vi "Compute Spot Pattern v2.vi"(0 "Images Dest":T1, 2 "Pattern Definition":T4={"X pitch"=20.0, "rotation"=0.0, "Center H"=0.0, "Center V"=0.0, "# Spots H"=8, "# Spots V"=8, "Spot size"=20.0, "ref_spot _dark"=FALSE, "Exact Phase Formula"=TRUE, "phase_wrap_pos"=TRUE, "Set Focus (mm)"=30.0, "phase_max"=4.0, "phase_factor"=65, "Steer LW"=0, "Steer vmax"=0, "phase_wrap_neg"=TRUE, "steer_horiz"=TRUE, "steer_pad"=0, "steer_only"=FALSE, "Wavelength"=628.0, "Y pitch"=0.0, "python"=FALSE, "test_pattern"=FALSE, "grid"=FALSE, "dark_all"=FALSE, "Xm_str"="21.72,  44.87,  68.20,  91.45, 114.72, 137.87, 160.97, 184.04", "Ym_str"="21.72,  44.87,  68.20,  91.45, 114.72, 137.87, 160.97, 184.04", "ref_spot"=0, "stretch"=FALSE} {"ref_spot" min=0 max=500 step=1 format="%#.0f"; "Y pitch" min=0.0 max=100.0 format="%.2g"; "Wavelength" min=0.0 max=500.0 format="%^#.3e"; "steer_pad" min=0 max=500 step=1 format="%#.0f"; "Steer LW" max=500; "phase_max" min=0.0 max=500.0 format="%#.3f"; "Set Focus (mm)" min=0.0 max=500.0 format="%#.3g"; "Spot size" min=1.0 format="%.2g"; "# Spots V" min=1 step=1; "# Spots H" min=1 step=1; "Center V" format="%.2f"; "Center H" format="%.2f"; "rotation" min=-90.0 max=90.0 format="%.2g"; "X pitch" min=0.0 max=100.0 format="%.2g"}, 3 "error in":errorcluster) -> (6 "Images Out":T1, 7 "Focal Distances":T3 {"fUser" format="%#.1g"; "fDiff" format="%#.1g"; "fFresnel" format="%#.1g"; "fWrap" format="%#.1g"}, 8 "ticks":u32, 9 "error out":errorcluster)   [LabVIEW 2011]
uses:
  Periodic Spot Pattern Parameters.ctl
  LCOS Images.ctl
  <vilib>/vision/Image Controls.llb/IMAQ Image.ctl
  Periodic Spot Pattern Parameters2.ctl
panel:
  out "last_xspot":i32
  out "first_xspot":i32
  out "pattern spotborder":dbl
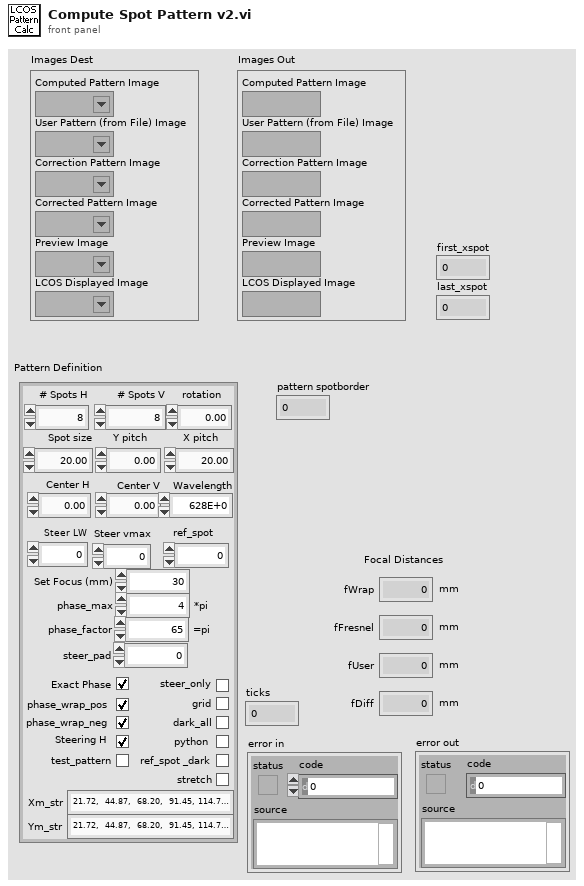
[diagram p1: front panel]
types:
  T1 = typedef "LCOS Images.ctl" = cluster{"Computed Pattern Image":T2, "User Pattern (from File) Image":T2, "Correction Pattern Image":T2, "Corrected Pattern Image":T2, "Preview Image":T2, "LCOS Displayed Image":T2}
  T2 = typedef "IMAQ Image.ctl" = refnum<image>
  T3 = cluster{"fWrap":dbl[unit], "fFresnel":dbl[unit], "fDiff":dbl[unit], "fUser":dbl[unit]}
  T4 = typedef "Periodic Spot Pattern Parameters.ctl" = cluster{"X pitch":dbl, "rotation":dbl, "Center H":dbl, "Center V":dbl, "# Spots H":u32, "# Spots V":u32, "Spot size":dbl, "ref_spot _dark":bool, "Exact Phase Formula":bool, "phase_wrap_pos":bool, "Set Focus (mm)":dbl, "phase_max":dbl, "phase_factor":u8, "Steer LW":u32, "Steer vmax":u8, "phase_wrap_neg":bool, "steer_horiz":bool, "steer_pad":i64, "steer_only":bool, "Wavelength":dbl, "Y pitch":dbl, "python":bool, "test_pattern":bool, "grid":bool, "dark_all":bool, "Xm_str":string, "Ym_str":string, "ref_spot":i64, "stretch":bool}
  T5 = typedef "Periodic Spot Pattern Parameters2.ctl" = dbl
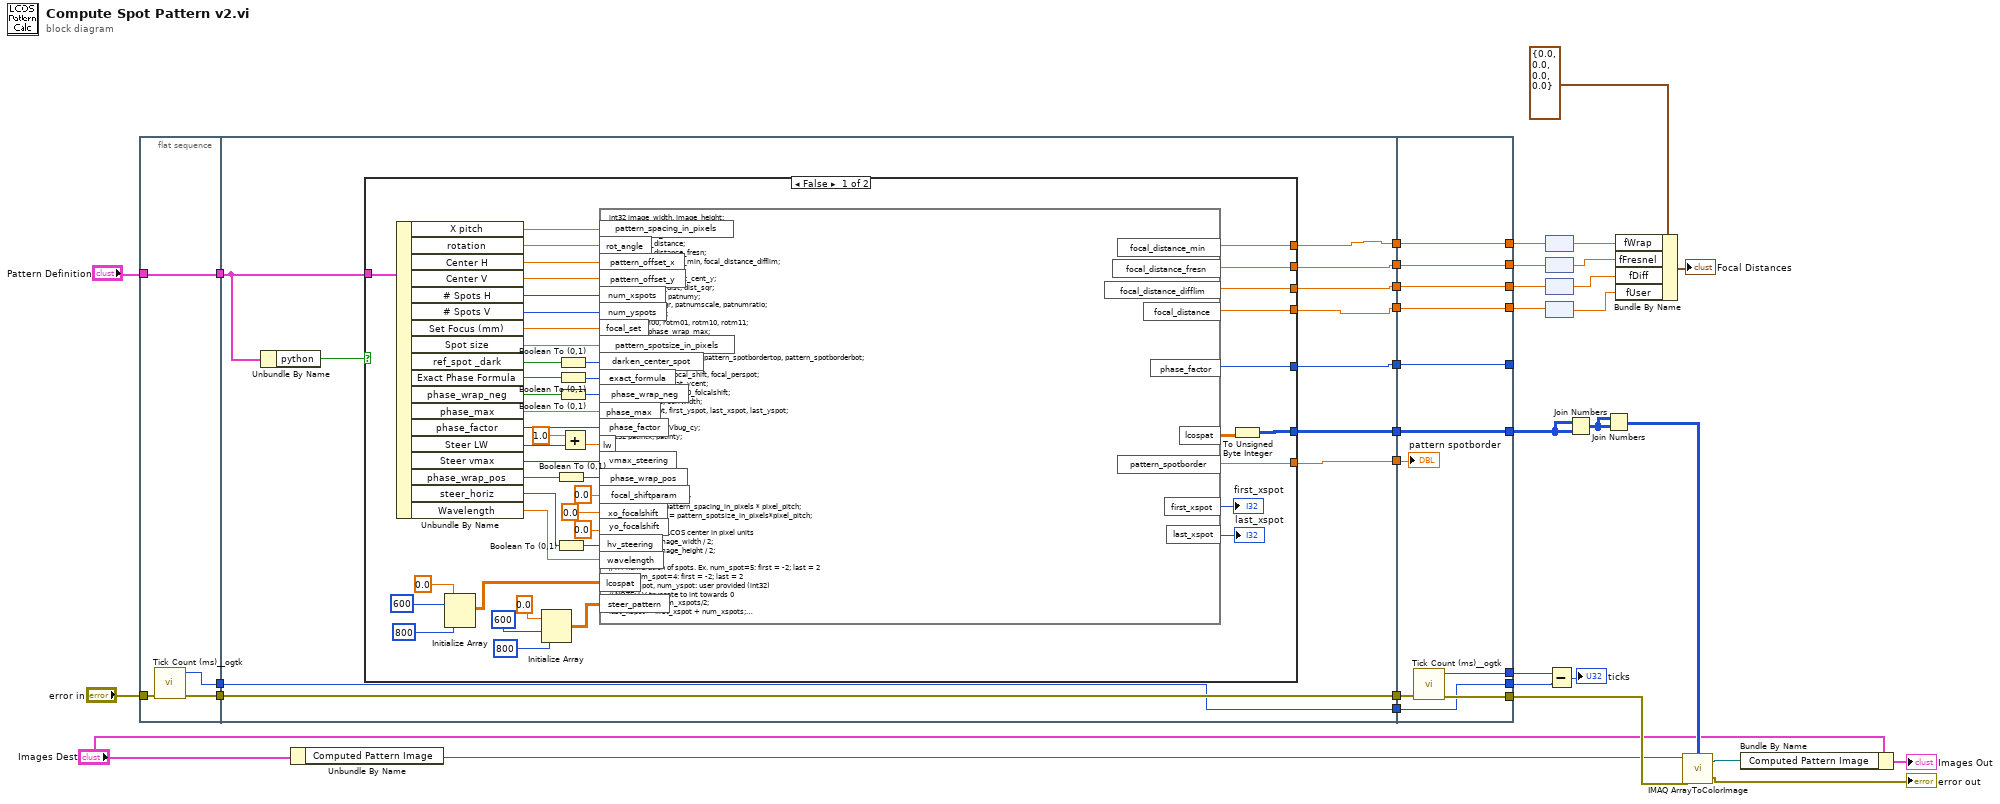
[diagram p0: block diagram]
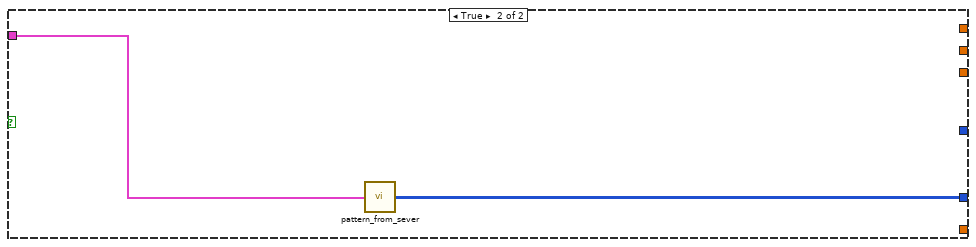
[diagram p2: hidden frame]
diagram:
  n1 = flat-sequence {
    tunnel: "error in" -> [w39]
    tunnel: "Pattern Definition" -> [w40]
    tunnel: [w40] -> w25
    tunnel: [w38] -> w24
    tunnel: [w37] -> w15
    tunnel: w25 -> [w43]
    tunnel: w24 -> [w51]
    tunnel: [w49] -> w22
    tunnel: [w48] -> w21
    tunnel: [w47] -> w20
    tunnel: [w46] -> w19
    tunnel: [w41] -> w18
    tunnel: [w51] -> w17
    tunnel: [w50] -> w16
    tunnel: w15 -> [w50]
    tunnel: [w45] -> w6
    tunnel: [w44] -> w1
    tunnel: [w101] -> w9
    tunnel: [w108] -> w30
    tunnel: [w109] -> w31
    tunnel: [w110] -> w32
    tunnel: [w111] -> w34
    tunnel: w22 -> [w111]
    tunnel: w21 -> [w110]
    tunnel: w20 -> [w109]
    tunnel: w19 -> [w108]
    tunnel: w18 -> [w101]
    tunnel: w17 -> [w107]
    tunnel: [w106] -> w11
    tunnel: w16 -> [w104]
    tunnel: [w105] -> w14
    tunnel: [w104] -> w13
    tunnel: [w103] -> _
    tunnel: w6 -> [w103]
    tunnel: w1 -> [w102]
    frame #0 {
      n2 = call <userlib>:"Tick Count (ms)__ogtk.vi"("error in (no error)"=w39) -> ("error out"=w38:errorcluster, "millisecond timer value"=w37:u32)  [unwired: 9 in]
    }
    frame #1 {
      n3 = Unbundle By Name(w43) -> ("python"=w42:bool)
      n4 = case shown="False" w42 {
        tunnel: [w68 _] -> w49
        tunnel: [w67 _] -> w48
        tunnel: [w66 _] -> w47
        tunnel: [w65 _] -> w46
        tunnel: [w64 _] -> w45
        tunnel: [w58 w99] -> w41
        tunnel: [w63 _] -> w44
        tunnel: w43 -> [w62 w100]
        frame False {
          n5 = Unbundle By Name(w62) -> ("X pitch"=w98:dbl, "rotation"=w97:dbl, "Center H"=w96:dbl, "Center V"=w95:dbl, "# Spots H"=w94:u32, "# Spots V"=w93:u32, "Set Focus (mm)"=w88:dbl, "Spot size"=w87:dbl, "ref_spot _dark"=w86:bool, "Exact Phase Formula"=w84:bool, "phase_wrap_neg"=w82:bool, "phase_max"=w80:dbl, "phase_factor"=w79:u8, "Steer LW"=w78:u32, "Steer vmax"=w77:u8, "phase_wrap_pos"=w52:bool, "steer_horiz"=w54:bool, "Wavelength"=w53:dbl)
          n6 = Initialize Array(0.0 ("element"), 600 ("dimension size"), 800 ("dimension size")) -> (w89:dbl[][])
          n7 = Initialize Array(0.0 ("element"), 600 ("dimension size"), 800 ("dimension size")) -> (w73:dbl[][])
          n8 = Boolean To (0,1)(Boolean=w52) -> (0, 1=w72:i16)
          n9 = Boolean To (0,1)(Boolean=w54) -> (0, 1=w69:i16)
          n10 = Boolean To (0,1)(Boolean=w86) -> (0, 1=w85:i16)
          n11 = Boolean To (0,1)(Boolean=w84) -> (0, 1=w83:i16)
          n12 = Boolean To (0,1)(Boolean=w82) -> (0, 1=w81:i16)
          n13 = Add(x=T5 1.0, y=w78) -> (x+y=w61:T5)
          n14 = formula code="int32 image_width, image_height;\nfloat64 pixel_pitch;\nfloat64 pattern_pitch;\nfloat64 focal_distance;\nfloat64 focal_distance_fresn;\nfloat64 focal_distance_min, focal_distance_difflim;\nfloat64 cos_theta;\nfloat64 pat_cent_x, pat_cent_y;\nfloat64 x_dist, y_dist, dist_sqr;\nfloat64 patnumx, patnumy;\nfloat64 patnumsqr, patnumscale, patnumratio;\nfloat64 rotx, roty;\nfloat64 rotm00, rotm01, rotm10, rotm11;\nfloat64 val, phase_wrap_max;\nfloat64 pattern_spotsize;\nfloat64 patnumx_frac, patnumy_frac;\nfloat64 pattern_spotborder, pattern_spotbordertop, pattern_spotborderbot;\nfloat64 quadratic_adj;\nfloat64 wrap_dist, focal_shift, focal_perspot;\nfloat64 pat_xcent, pat_ycent;\nfloat64 x0_folcalshift, y0_folcalshift;\nint32 corrheight, corrwidth;\nint32 first_xspot, first_yspot, last_xspot, last_yspot;\nint32 x, y, d;\nint32 LVbug_cx, LVbug_cy;\nint32 patintx, patinty;\n\n// USER CONSTANTS\nimage_width = 800;\nimage_height = 600;\npixel_pitch = 20e-6;\n\n// Pattern size/geometry\npattern_pitch = pattern_spacing_in_pixels * pixel_pitch;\npattern_spotsize = pattern_spotsize_in_pixels*pixel_pitch;\n\n// Coordinates of LCOS center in pixel units\npat_cent_x = image_width / 2;\npat_cent_y = image_height / 2;\n\n// XY numeration of spots. Ex. num_spot=5: first = -2; last = 2\n//\t\t\t\t\t\t\t   num_spot=4: first = -2; last = 2\n// num_xspot, num_yspot: user provided (int32)\n// NOTE: LV truncate to int towards 0\nfirst_xspot = -num_xspots/2;\nlast_xspot = first_xspot + num_xspots;\nfirst_yspot = -num_yspots/2;\nlast_yspot = first_yspot + num_yspots;\nLVbug_cx = 0;\nLVbug_cy = 0;\n\n// - - - SPOT BORDER - - - (useful when spot_size , spot_pitch)\n// Spot border width in percentage of pattern_pitch (or pattern_pitch units)\npattern_spotborder = 0.5*(1 - pattern_spotsize/pattern_pitch);\n// Border start coordinate on top/bottom in pattern_pitch units\npattern_spotbordertop = 0.5 - pattern_spotborder;\npattern_spotborderbot = -0.5 + pattern_spotborder;\n\n// Rescale pattern translation/rotation in standard units\npattern_offset_x *= pixel_pitch;                   // mod XM\npattern_offset_y *= pixel_pitch;                  // mod XM\nrot_angle *= (pi/180);                                 // mod XM\n\n// Use user-provided focal distance\nfocal_distance = focal_set * 1e-3;\n\n// Recenter odd numbered spots.\nif (num_xspots & 1) {\n\tpattern_offset_x -= 0.5*pattern_pitch * (1 - (num_xspots & 2));\n\tLVbug_cx = -(num_xspots & 2) / 2;\n}\nif (num_yspots & 1) {\n\tpattern_offset_y -= 0.5*pattern_pitch * (1 - (num_yspots & 2));\n\tLVbug_cy = -(num_yspots & 2) / 2;\n}\n\n// Prepare rotation matrix.\nrotm00 = cos(rot_angle);\nrotm01 = sin(rot_angle);\nrotm11 = rotm00;\nrotm10 = -rotm01;\n\n// Calculate pattern\nfor (y=0; y<image_height; y++) {\n\tfor (x=0; x<image_width; x++) {\n\t\t// Calculate pattern in rotated space.\n\t\t// rotx, roty: rotated&centered coordinates in pixel units\n\t\trotx = rotm00 * (x-pat_cent_x) + rotm01 * (y-pat_cent_y);\n\t\troty = rotm10 * (x-pat_cent_x) + rotm11 * (y-pat_cent_y);\n\n\t\t// Square distance from pattern center in pattern_pitch (spot number) units\n\t\tpatnumsqr = (pixel_pitch**2)*(rotx**2 + roty**2)/(pattern_pitch**2);\n\n\t\t// Rotated&centered coordinates in spot-number units\n\t\tpatnumx = (rotx*pixel_pitch-pattern_offset_x)/pattern_pitch;\n\t\tpatnumy = (roty*pixel_pitch-pattern_offset_y)/pattern_pitch;\n\n\t\t// Center of current spot in meters\n\t\tpat_xcent = pattern_pitch*(floor(patnumx) + 0.5);\n\t\tpat_ycent = pattern_pitch*(floor(patnumy) + 0.5);\n\n\t\t// Coordinates relative to the spot center in spot-number units\n\t\tpatnumx_frac = patnumx - (floor(patnumx) + 0.5);\n\t\tpatnumy_frac = patnumy - (floor(patnumy) + 0.5);\n\n\t\t// If this spot number is in the range.\n\t\tif ((patnumx >= first_xspot) && (patnumx < last_xspot) &&\n\t\t\t(patnumy >= first_yspot) && (patnumy < last_yspot) &&\n\t\t\t(patnumx_frac >= pattern_spotborderbot) &&\n\t\t\t(patnumx_frac <= pattern_spotbordertop) &&\n\t\t\t(patnumy_frac >= pattern_spotborderbot) &&\n\t\t\t(patnumy_frac <= pattern_spotbordertop) ) {\n\n\t\t\tx0_folcalshift = pattern_pitch*(floor(patnumx)-xo_focalshift);\n\t\t\ty0_folcalshift = pattern_pitch*(floor(patnumy)+yo_focalshift);\n\t\t\tfocal_shift = focal_shiftparam*(x0_folcalshift**2 + y0_folcalshift**2);\n\t\t\tfocal_perspot = focal_distance + focal_shift;\n\n\t\t\tif (darken_center_spot &&\n\t\t\t\tpatnumx < 1+LVbug_cx && patnumx > LVbug_cx &&\n\t\t\t\tpatnumy < 1+LVbug_cy && patnumy > LVbug_cy) {\n\t\t\t\tlcospat[y][x] = 0;\n\t\t\t\tcontinue;\n\t\t\t}\n\n\t\t\t// Coordinates relative to the spot center in meters\n\t\t\tx_dist = pattern_pitch * patnumx_frac;\n\t\t\ty_dist = pattern_pitch * patnumy_frac;\n\n\t\t\tdist_sqr = x_dist*x_dist + y_dist*y_dist;\n\n\t\t\tif (exact_formula) {\n\t\t\t\tcos_theta = cos(atan(sqrt(dist_sqr)/focal_perspot));\n\t\t\t\tlcospat[y][x] = phase_max - 1e-6 - (2/wavelength) * (1-cos_theta) * sqrt(dist_sqr + focal_perspot**2);\n\t\t\t}\n\t\t\telse\n\t\t\t\tlcospat[y][x] = phase_max - 1e-6 - dist_sqr / (wavelength*focal_distance);\n\t\t}\n\t\telse {\n\t\t// Make unused area plane wave, to be filtered out by pindot.\n\t\tlcospat[y][x] = 0;\n\t\t}\n\t}\n}\n\n// Steering specular reflection out of the field of view\nfor (y=0; y<image_height; y++) {\n\tfor (x=0; x<image_width; x++) {\n\t\td = hv_steering ? y: x;\n\t\tsteer_pattern[y][x] = (d - lw*floor(d/lw))/(lw-1)*vmax_steering;\n\t}\n}\n\n// Map to greyscale values\nfor (y=0; y<image_height; y++) {\n\tfor (x=0; x<image_width; x++) {\n\t\tval = lcospat[y][x];\n\n\t\t// Set the outside of the pattern for beam steering\n\t\tif ((val == 0) && (lw > 1))\n\t\t\tval = steer_pattern[y][x] / phase_factor;\n\n        // compute smallest multiple of 2 contained in phase_max\n        if (phase_wrap_neg || phase_wrap_pos) {\n            if (phase_max <= 2)\n                phase_wrap_max = 2;\n            else\n                phase_wrap_max = floor(phase_max / 2) * 2;\n        }\n\n\t\t// Wrap negative phase values or set them to 0\n\t\tif ((!phase_wrap_neg) && (val < 0))\n\t\t\tval = 0;\n        else if (phase_wrap_neg) {\n\t\t\tif (val < 0) {\n                // modulus of val over phase_wrap_max\n\t\t\t\tval -= floor(val/phase_wrap_max) * phase_wrap_max;\n            }\n\t\t}\n\n        // Wrap positive phase values above 2*pi\n        if (phase_wrap_pos) {\n            if (val > 2) {\n                // modulus of val over phase_wrap_max\n                val -= floor(val/phase_wrap_max) * phase_wrap_max;\n            }\n        }\n\n\t\t// Map PI to correct greyscale value.\n\t\tval = val * phase_factor;\n\n\t\tlcospat[y][x] = val;\n\t}\n}"("pattern_spacing_in_pixels"=w98, "rot_angle"=w97, "pattern_offset_x"=w96, "pattern_offset_y"=w95, "num_xspots"=w94, "num_yspots"=w93, "lcospat"=w89, "focal_set"=w88, "pattern_spotsize_in_pixels"=w87, "darken_center_spot"=w85, "exact_formula"=w83, "phase_wrap_neg"=w81, "phase_max"=w80, "phase_factor"=w79, "lw"=w61, "vmax_steering"=w77, "steer_pattern"=w73, "phase_wrap_pos"=w72, "focal_shiftparam"=T5 0.0 ("input variable"), "xo_focalshift"=T5 0.0 ("input variable"), "yo_focalshift"=T5 0.0 ("input variable"), "hv_steering"=w69, "wavelength"=w53) -> ("focal_distance_min"=w68:dbl, "focal_distance_fresn"=w67:dbl, "focal_distance_difflim"=w66:dbl, "focal_distance"=w65:dbl, "lcospat"=w59:dbl[][], "phase_factor"=w64:u8, "pattern_spotborder"=w63:dbl, "first_xspot"=→"first_xspot":i32, "last_xspot"=→"last_xspot":i32)
          n15 = To Unsigned Byte Integer(number=w59) -> (unsigned 8bit integer=w58:u8[][])
        }
        frame True {
          n16 = call "pattern_from_sever.vi"("Pattern Definition"=w100) -> ("data out"=w99:u8[][])
        }
      }
    }
    frame #2 {
      n17 = call <userlib>:"Tick Count (ms)__ogtk.vi"("error in (no error)"=w107) -> ("error out"=w106:errorcluster, "millisecond timer value"=w105:u32)  [unwired: 9 in]
      "pattern spotborder" <- w102
    }
  }
  n18 = Unbundle By Name("Images Dest") -> ("Computed Pattern Image"=w5:T2)
  n19 = node(w34) -> (w33:dbl[unit])
  n20 = node(w32) -> (w29:dbl[unit])
  n21 = node(w31) -> (w28:dbl[unit])
  n22 = node(w30) -> (w27:dbl[unit])
  n23 = Subtract(x=w14, y=w13) -> (x-y=→"ticks":u32)
  n24 = Join Numbers(hi=w9, lo=w9) -> ((hi.lo)=w8:u16[][])
  n25 = Join Numbers(hi=w8, lo=w8) -> ((hi.lo)=w7:u32[][])
  n26 = Bundle By Name(cluster=T3 {"fWrap"=0.0, "fFresnel"=0.0, "fDiff"=0.0, "fUser"=0.0} ("Focal Distances"), "fWrap"=w33, "fFresnel"=w29, "fDiff"=w28, "fUser"=w27) -> (→"Focal Distances":T3)
  n27 = call "IMAQ ArrayToColorImage"("Image Pixels (U32)"=w7, "Image"=w5, "error in (no error)"=w11) -> ("Image Out"=w2:T2, "error out"=→"error out":errorcluster)  [unwired: 2 in]
  n28 = Bundle By Name(cluster="Images Dest", "Computed Pattern Image"=w2) -> (→"Images Out":T1)
